vi "AOC1_Part1.vi"() -> ()   [LabVIEW 2015]
panel:
  out "Floor Number":i32
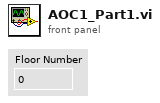
[diagram p1: front panel]
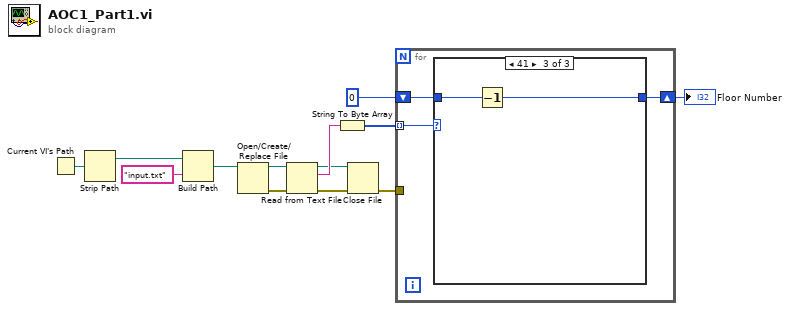
[diagram p0: block diagram]
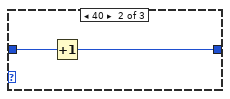
[diagram p3: hidden frame]
diagram:
  n1 = Current VI's Path() -> (path=w11:path)
  n2 = Strip Path(path=w11) -> (stripped path=w10:path)  [unwired: 1 out]
  n3 = Build Path(base path=w10, name or relative path="input.txt") -> (appended path=w8:path)
  n4 = Open/Create/Replace File(file path (use dialog)=w8) -> (refnum out=w12:refnum<file>, error out=w13:errorcluster)  [unwired: 5 in, 1 out]
  n5 = Read from Text File(file (use dialog)=w12, error in=w13) -> (refnum out=w5:refnum<file>, text=w7:string, error out=w6:errorcluster)  [unwired: 2 in, 1 out]
  n6 = String To Byte Array(string=w7) -> (unsigned byte array=w4:u8[])
  n7 = Close File(refnum=w5, error in=w6) -> (error out=w3:errorcluster)  [unwired: 1 out]
  n8 = for {
    tunnel: w4 -> [w16] mode=indexing
    tunnel: w3 -> [_]
    shift-right: [w14] -> w1
    shift-left: 0 -> [w15]
    n9 = case shown="41" w16 {
      tunnel: w15 -> [w17 w19 w21]
      tunnel: [w17 w18 w20] -> w14
      frame Default {
      }
      frame 40 {
        n10 = Increment(x=w19) -> (x+1=w18:i32)
      }
      frame 41 {
        n11 = Decrement(x=w21) -> (x-1=w20:i32)
      }
    }
  }
  "Floor Number" <- w1
